vi "Plot Codes.vi"() -> ()   [LabVIEW 2012, in "Error Logger.lvclass"]
uses:
  Error Logger.lvclass
panel:
  out "Array 2":i32[](array[numeric])
  out "Array":timestamp[](array[timestamp])
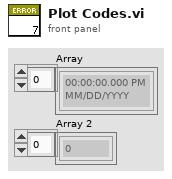
[diagram p1: front panel]
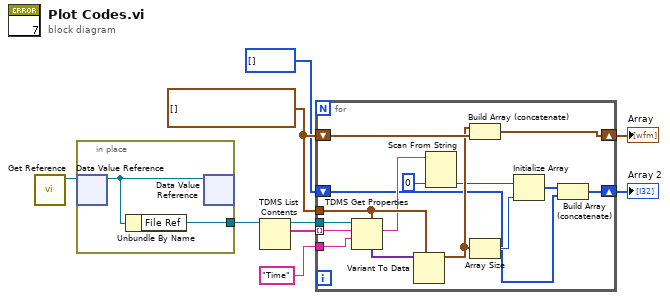
[diagram p0: block diagram]
diagram:
  w4 = timestamp[] []
  n1 = call "Get Reference.vi"() -> ("DVR"=w9:refnum<data-value>)  [unwired: 10 in, 1 out]
  n2 = in-place {
    in-place-border: [w10] -> w8
    n3 = in-place-dvr #1(w9) -> (w11:refnum<class "Error Logger.lvclass">)  [unwired: 1 out]
    n4 = Unbundle By Name(w11) -> ("File Ref"=w10:refnum<k34>)
    n5 = in-place-dvr #1(w11) -> ()  [unwired: 2 out]
  }
  n6 = TDMS List Contents(7:w8) -> (2:w7:string[], 3:w5:refnum<k34>)  [unwired: 2 in, 2 out]
  n7 = for {
    tunnel: w7 -> [w26] mode=indexing
    tunnel: w4 -> [w24]
    tunnel: "Time" -> [w13]
    tunnel: w5 -> [w25]
    shift-right: [w23] -> w3
    shift-left: w4 -> [w22]
    shift-right: [w15] -> w1
    shift-left: i32[] [] -> [w14]
    n8 = TDMS Get Properties(5:w24, 9:w13, 10:w26, 11:w25) -> (2:w21:string, 4:w12:variant[])  [unwired: 2 in, 4 out]
    n9 = Variant To Data(type=w24, Variant=w12) -> (data=w19:timestamp[])  [unwired: 1 in, 1 out]
    n10 = Scan From String(input string=w21, default 1=0) -> (output 1=w17:i32)  [unwired: 3 in, 3 out]
    n11 = Build Array (concatenate)(w19, w22) -> (w23:timestamp[])
    n12 = Array Size(array=w19) -> (size(s)=w18:i32)
    n13 = Initialize Array(w17, w18) -> (w16:i32[])
    n14 = Build Array (concatenate)(w16, w14) -> (w15:i32[])
  }
  "Array" <- w3
  "Array 2" <- w1
